vi "_GenerateExecuteExpression.vi"(6 "first call?":bool, 8 "error in (no error)":errorcluster, 9 "States":i32[](array[numeric]), 10 "StateNames":string[](array[string]), 11 "RulesMap":variant[](array[variant])) -> (0 "error out":errorcluster, 1 "condition":string[](array[string]), 2 "exps":cluster{"Tag":string, "formula":string}[](array[cluster]))   [LabVIEW 2017, in "TagDB RefManager.lvlib"]
uses:
  TagDB RefManager.lvlib
  Typedef/RefMgr-StateChangeType.ctl
  Typedef/RefMgr-Logic-State.ctl
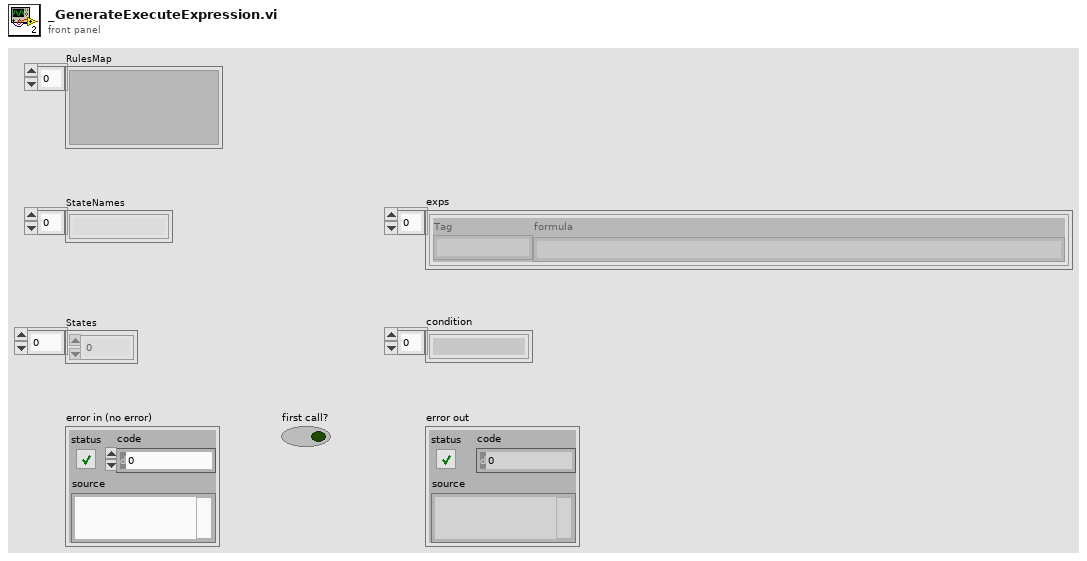
[diagram p1: front panel]
types:
  T1 = typedef "TagDB RefManager.lvlib/RefMgr-Logic-State.ctl" = cluster{"StateName":string, "StateValue":i32, "Type":T2, "Calcs":cluster{"Tag":string, "Exp":string}[]}
  T2 = typedef "TagDB RefManager.lvlib/RefMgr-StateChangeType.ctl" = enum16{"0 - 进入", "1 - 等于", "2 - 退出"}
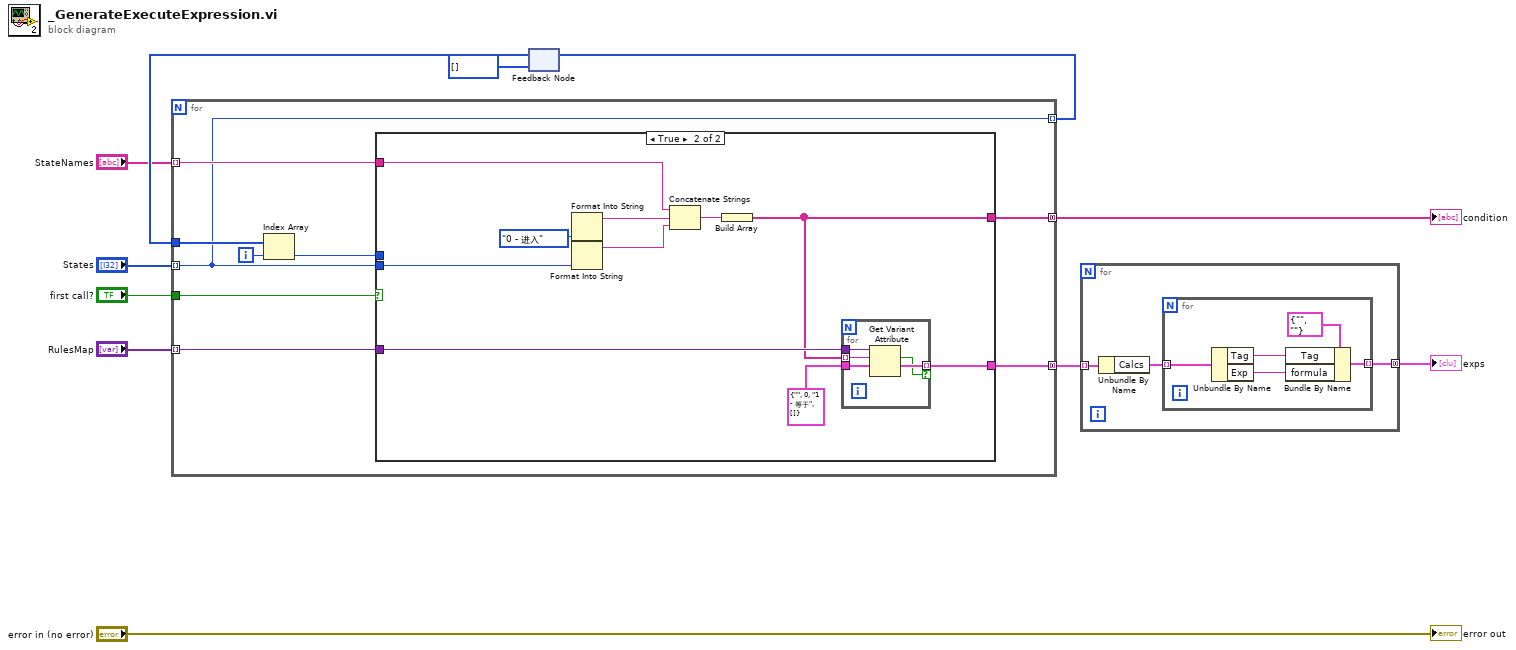
[diagram p0: block diagram]
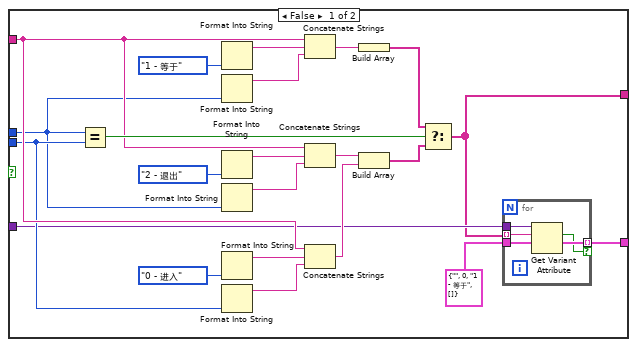
[diagram p2: hidden frame]
diagram:
  n1 = feedback #1(i32[] []) -> (w8:i32[])
  n2 = for {
    tunnel: "StateNames" -> [w19] mode=indexing
    tunnel: [w12] -> w7 mode=indexing
    tunnel: w8 -> [w20]
    tunnel: [w17] -> w11 mode=concatenating
    tunnel: "RulesMap" -> [w18] mode=indexing
    tunnel: "first call?" -> [w14]
    tunnel: [w13] -> w3 mode=concatenating
    tunnel: "States" -> [w12] mode=indexing
    i -> [w15]
    n3 = Index Array(array=w20, index=w15) -> (element=w16:i32)
    n4 = case shown="True" w14 {
      tunnel: w19 -> [w30 w54]
      tunnel: w12 -> [w29 w53]
      tunnel: w18 -> [w25 w51]
      tunnel: [w23 w49] -> w17
      tunnel: w16 -> [w22 _]
      tunnel: [w21 w48] -> w13
      frame False {
        n5 = Equal?(x=w22, y=w29) -> (x = y?=w42:bool)
        n6 = Format Into String(RefMgr-StateChangeType."1 - 等于" ("Type")) -> (resulting string=w40:string)  [unwired: 3 in, 1 out]
        n7 = Format Into String(w22) -> (resulting string=w39:string)  [unwired: 3 in, 1 out]
        n8 = Format Into String(RefMgr-StateChangeType."2 - 退出" ("Type")) -> (resulting string=w34:string)  [unwired: 3 in, 1 out]
        n9 = Format Into String(w22) -> (resulting string=w35:string)  [unwired: 3 in, 1 out]
        n10 = Format Into String(RefMgr-StateChangeType."0 - 进入" ("Type")) -> (resulting string=w33:string)  [unwired: 3 in, 1 out]
        n11 = Format Into String(w29) -> (resulting string=w32:string)  [unwired: 3 in, 1 out]
        n12 = Concatenate Strings(w30, w40, w39) -> (w37:string)
        n13 = Concatenate Strings(w30, w34, w35) -> (w28:string)
        n14 = Concatenate Strings(w30, w33, w32) -> (w27:string)
        n15 = Build Array(w37) -> (w41:string[])
        n16 = Build Array(w28, w27) -> (w26:string[])
        n17 = Select(t=w41, s=w42, f=w26) -> (s? t:f=w21:string[])
        n18 = for {
          tunnel: w25 -> [w47]
          tunnel: w21 -> [w46] mode=indexing
          tunnel: T1 {"StateName"="", "StateValue"=0, "Type"=enum."1 - 等于", "Calcs"=[]} ("Cluster") -> [w45]
          tunnel: [w44] -> w23 mode=indexing if=w43
          n19 = Get Variant Attribute(Variant=w47, name=w46, default value (empty Variant)=w45) -> (found=w43:bool, value=w44:T1)  [unwired: 1 in, 2 out]
        }
      }
      frame True {
        n20 = Format Into String(RefMgr-StateChangeType."0 - 进入" ("Type")) -> (resulting string=w57:string)  [unwired: 3 in, 1 out]
        n21 = Format Into String(w53) -> (resulting string=w56:string)  [unwired: 3 in, 1 out]
        n22 = Concatenate Strings(w54, w57, w56) -> (w52:string)
        n23 = Build Array(w52) -> (w48:string[])
        n24 = for {
          tunnel: w51 -> [w62]
          tunnel: w48 -> [w61] mode=indexing
          tunnel: T1 {"StateName"="", "StateValue"=0, "Type"=enum."1 - 等于", "Calcs"=[]} ("Cluster") -> [w60]
          tunnel: [w59] -> w49 mode=indexing if=w58
          n25 = Get Variant Attribute(Variant=w62, name=w61, default value (empty Variant)=w60) -> (found=w58:bool, value=w59:T1)  [unwired: 1 in, 2 out]
        }
      }
    }
  }
  "condition" <- w3
  n26 = feedback-in #1(w7) -> ()
  n27 = for {
    tunnel: w11 -> [w65] mode=indexing
    tunnel: [w63] -> w4 mode=concatenating
    n28 = Unbundle By Name(w65) -> ("Calcs"=w64:cluster{"Tag":string, "Exp":string}[])
    n29 = for {
      tunnel: w64 -> [w70] mode=indexing
      tunnel: [w68] -> w63 mode=indexing
      n30 = Unbundle By Name(w70) -> ("Tag"=w67:string, "Exp"=w69:string)
      n31 = Bundle By Name(cluster=cluster{"Tag":string, "formula":string} {"Tag"="", "formula"=""} ("type"), "Tag"=w67, "formula"=w69) -> (w68:cluster{"Tag":string, "formula":string})
    }
  }
  "exps" <- w4
  "error out" <- "error in (no error)"
